vi "subvi_min_max_timer_analyser1.vi"(8 "Timer Functions":T1=enum."Timed Out & Reset", 9 "Minimum Threshold Time (ms)":u32=100, 10 "Manual Reset":bool=TRUE, 11 "Maximum Threshold Time (ms)":u32=100) -> (1 "Elapsed Time (ms)":u32, 3 "Timed Out?":bool=TRUE)   [LabVIEW 2014]
doc: "Timed Out: returns True when the Threshold Time (ms) is reached.\nTimed Out & Reset: returns True when the Threshold Time (ms) is reached and resets the Start Time so that the function will keep on timing out when reaching the threshold time.\nInitialise: initialises the Start Time. \nReset: resets the Start Time to zero."
uses:
  Timer/typedef_timer.ctl
panel:
  out "Minimum Threshold Time (ms)":u32
  out "Maximum Threshold Time (ms)":u32
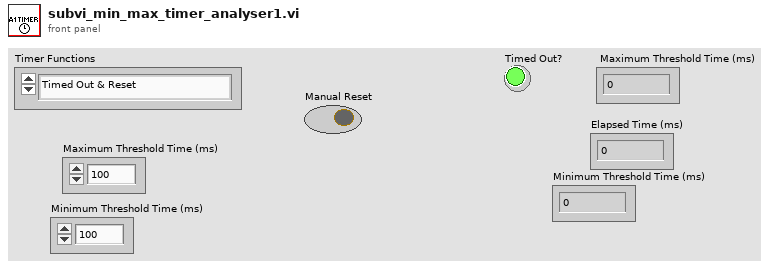
[diagram p1: front panel]
types:
  T1 = typedef "typedef_timer.ctl" = enum16{"Inside Time Window & Manual Reset", "Inside Time Window", "Reset", "Initialise", "Timed Out & Reset", "Timed Out"}
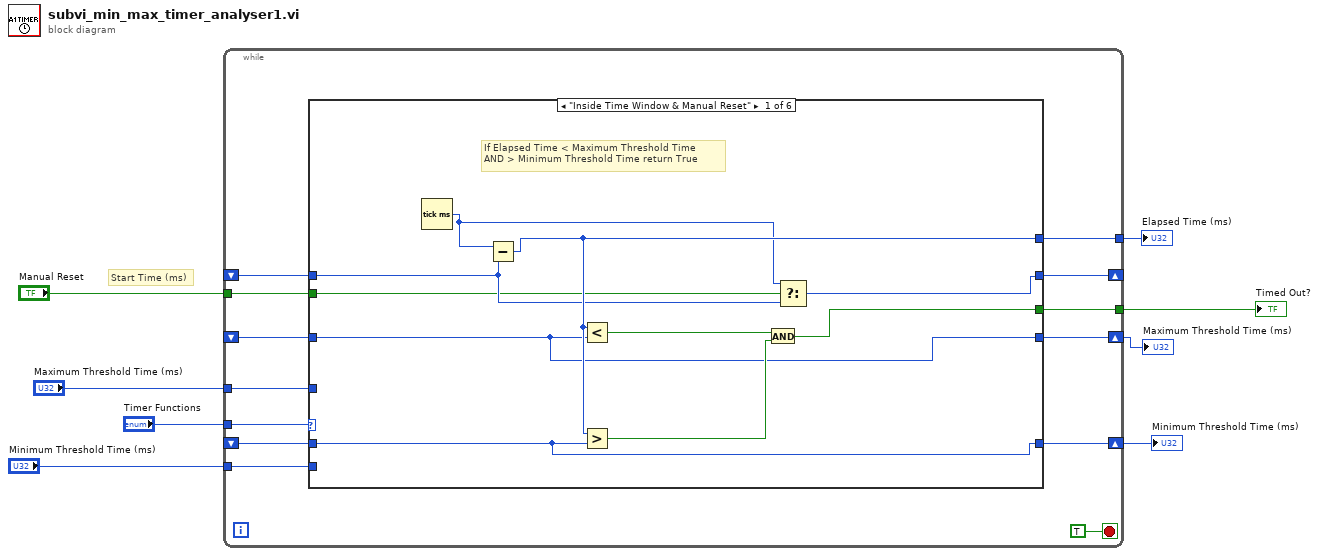
[diagram p0: block diagram]
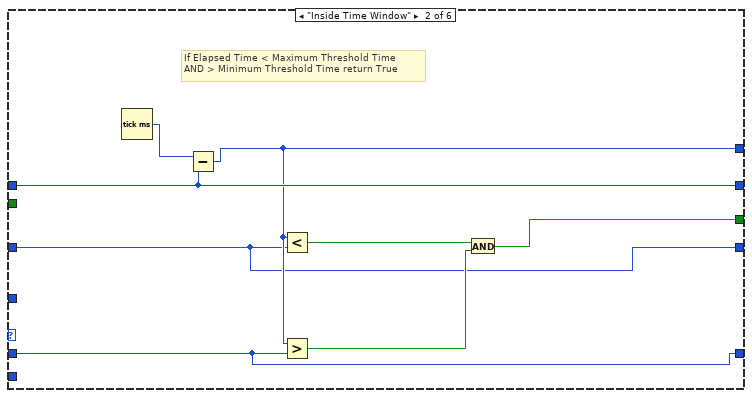
[diagram p2: hidden frame]
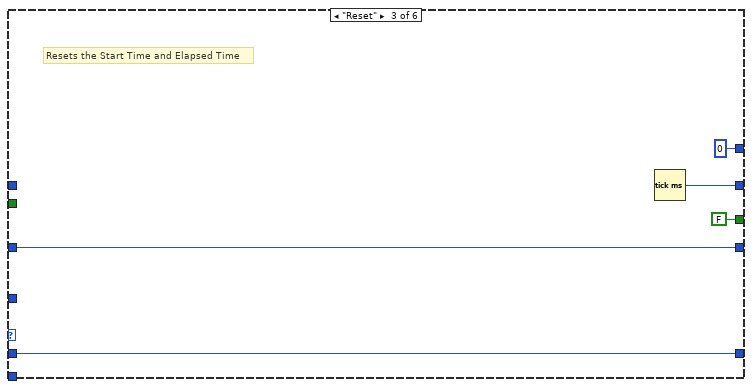
[diagram p3: hidden frame]
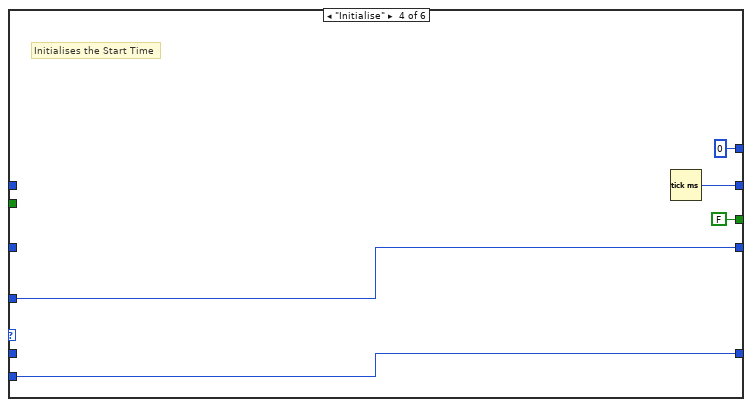
[diagram p4: hidden frame]
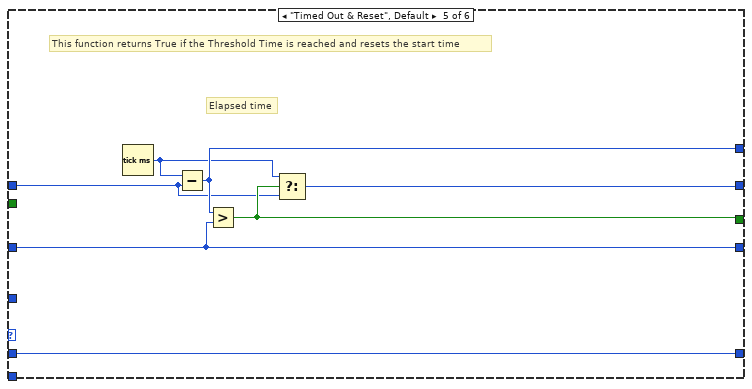
[diagram p5: hidden frame]
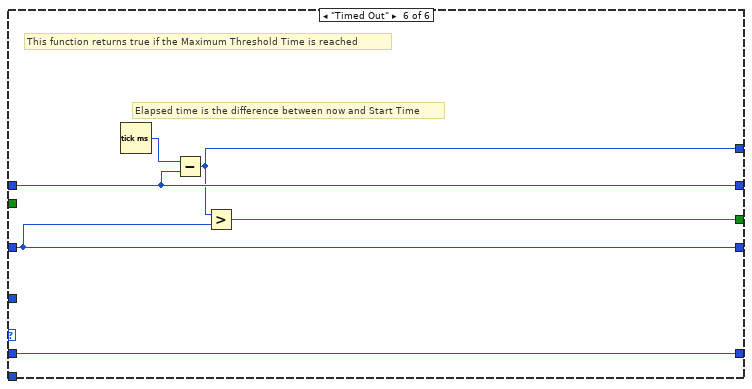
[diagram p6: hidden frame]
diagram:
  # "Start Time (ms)"
  n1 = while {
    tunnel: "Timer Functions" -> [w21]
    shift-right: [w18] -> _
    shift-left: _ -> [w20]
    shift-right: [w17] -> w5
    shift-left: _ -> [w19]
    tunnel: [w16] -> w7
    tunnel: "Maximum Threshold Time (ms)" -> [w14]
    tunnel: [w13] -> w4
    tunnel: "Minimum Threshold Time (ms)" -> [w12]
    shift-right: [w10] -> w2
    shift-left: _ -> [w11]
    tunnel: "Manual Reset" -> [w9]
    stop <- TRUE stop-if-true
    n2 = case shown="\"Inside Time Window & Manual Reset\"" w21 {
      tunnel: w20 -> [w24 w38 _ _ w53 w61]
      tunnel: w19 -> [w27 w33 w42 _ w56 w60]
      tunnel: [w22 w38 w44 w47 w51 w61] -> w18
      tunnel: [w27 w33 w42 w49 w56 w60] -> w17
      tunnel: [w28 w34 FALSE FALSE w54 w59] -> w16
      tunnel: w14 -> [_ _ _ w49 _ _]
      tunnel: [w31 w37 u32 0 u32 0 w55 w58] -> w13
      tunnel: w12 -> [_ _ _ w45 _ _]
      tunnel: w11 -> [w26 w32 w40 _ w50 w57]
      tunnel: [w26 w32 w40 w45 w50 w57] -> w10
      tunnel: w9 -> [w23 _ _ _ _ _]
      frame "Inside Time Window & Manual Reset" {
        # "If Elapsed Time < Maximum Threshold Time\nAND > Minimum Threshold Time return True"
        n3 = Tick Count (ms)() -> (millisecond timer value=w25:u32)
        n4 = Subtract(x=w25, y=w24) -> (x-y=w31:u32)
        n5 = Less?(x=w31, y=w27) -> (x < y?=w30:bool)
        n6 = Greater?(x=w31, y=w26) -> (0:w29:bool)
        n7 = And(x=w30, y=w29) -> (x .and. y?=w28:bool)
        n8 = Select(t=w25, s=w23, f=w24) -> (s? t:f=w22:u32)
      }
      frame "Inside Time Window" {
        # "If Elapsed Time < Maximum Threshold Time\nAND > Minimum Threshold Time return True"
        n9 = Tick Count (ms)() -> (millisecond timer value=w39:u32)
        n10 = Subtract(x=w39, y=w38) -> (x-y=w37:u32)
        n11 = Less?(x=w37, y=w33) -> (x < y?=w36:bool)
        n12 = Greater?(x=w37, y=w32) -> (0:w35:bool)
        n13 = And(x=w36, y=w35) -> (x .and. y?=w34:bool)
      }
      frame "Reset" {
        # "Resets the Start Time and Elapsed Time"
        n14 = Tick Count (ms)() -> (millisecond timer value=w44:u32)
      }
      frame "Initialise" {
        # "Initialises the Start Time"
        n15 = Tick Count (ms)() -> (millisecond timer value=w47:u32)
      }
      frame "Timed Out & Reset", Default {
        # "Elapsed time"
        # "This function returns True if the Threshold Time is reached and resets the start time"
        n16 = Tick Count (ms)() -> (millisecond timer value=w52:u32)
        n17 = Subtract(x=w52, y=w53) -> (x-y=w55:u32)
        n18 = Greater?(x=w55, y=w56) -> (0:w54:bool)
        n19 = Select(t=w52, s=w54, f=w53) -> (s? t:f=w51:u32)
      }
      frame "Timed Out" {
        # "Elapsed time is the difference between now and Start Time"
        # "This function returns true if the Maximum Threshold Time is reached"
        n20 = Tick Count (ms)() -> (millisecond timer value=w62:u32)
        n21 = Subtract(x=w62, y=w61) -> (x-y=w58:u32)
        n22 = Greater?(x=w58, y=w60) -> (0:w59:bool)
      }
    }
  }
  "Timed Out?" <- w7
  "Maximum Threshold Time (ms)" <- w5
  "Elapsed Time (ms)" <- w4
  "Minimum Threshold Time (ms)" <- w2
